vi "FGV_EventToSplashScreen.vi"(7 "Command":T1, 8 "error in (no error)":errorcluster) -> (0 "error out":errorcluster, 3 "ToSplashScreenEvent":refnum<user-event>)   [LabVIEW 2013]
uses:
  EnumFgvEventCommand.ctl
  ToSplashScreen.ctl
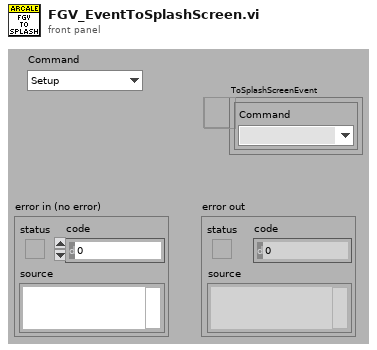
[diagram p1: front panel]
types:
  T1 = typedef "EnumFgvEventCommand.ctl" = enum16{"Setup", "Cleanup", "Get"}
  T2 = typedef "ToSplashScreen.ctl" = cluster{"Command":enum16{"Stop"}}
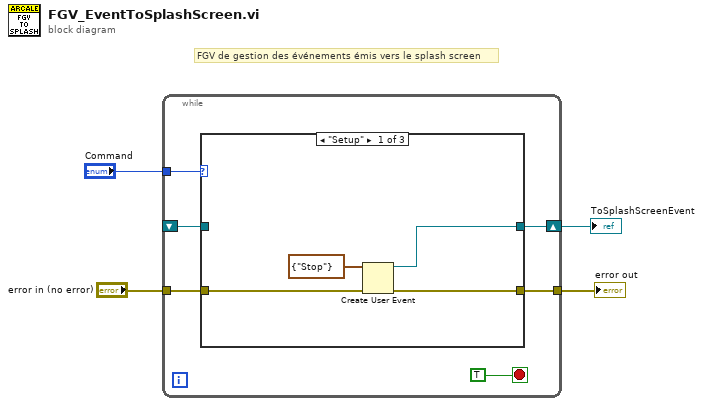
[diagram p0: block diagram]
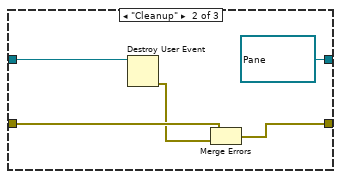
[diagram p2: hidden frame]
diagram:
  # "FGV de gestion des événements émis vers le splash screen"
  n1 = while {
    tunnel: "Command" -> [w10]
    tunnel: "error in (no error)" -> [w8]
    tunnel: [w7] -> w2
    shift-right: [w6] -> w1
    shift-left: _ -> [w5]
    stop <- TRUE stop-if-true
    n2 = case shown="\"Setup\"" w10 {
      tunnel: w8 -> [w14 w17 w20]
      tunnel: [w12 w15 w20] -> w7
      tunnel: [w11 refnum<user-event> refnum ("ToSplashScreen") w21] -> w6
      tunnel: w5 -> [_ w19 w21]
      frame "Setup" {
        n3 = Create User Event(user event datatype=T2 {"Command"=enum."Stop"} ("ToSplashScreen"), error in=w14) -> (user event=w11:refnum<user-event>, error out=w12:errorcluster)
      }
      frame "Cleanup" {
        n4 = Destroy User Event(user event=w19) -> (error out=w16:errorcluster)  [unwired: 1 in]
        n5 = Merge Errors(w17, w16) -> (w15:errorcluster)
      }
      frame "Get" {
      }
    }
  }
  "error out" <- w2
  "ToSplashScreenEvent" <- w1
